vi "missing_Peak.vi"() -> ()   [LabVIEW 2016]
panel:
  out "x+y":i32
  out "Numeric":i32
  out "element":i32
  out "size(s)":i32
  out "Phase 2":dbl[](array[numeric])
  out "Peak Locations 2":i32[](array[numeric])
  in  "Width":dbl format="%#_13g"
  in  "Phase":dbl[](array[numeric])=[0.5, 1.55, 0.7, 0.8, 0.2, 0.3]
  in  "Peak Locations":i32[](array[numeric])=[1, 3, 4, 5]
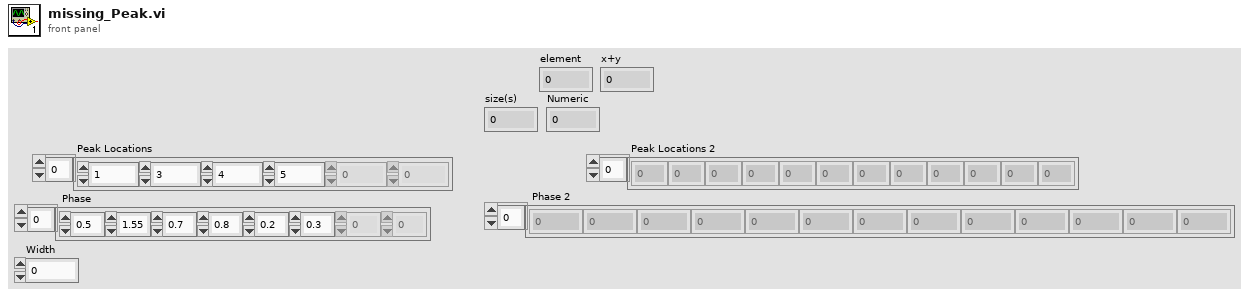
[diagram p1: front panel]
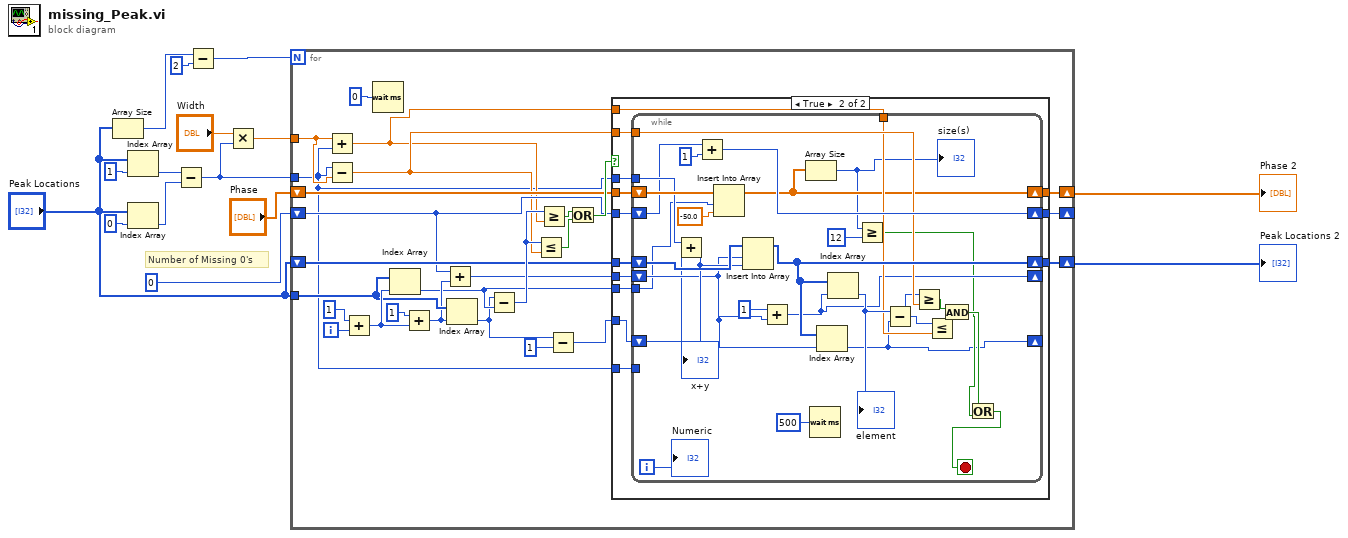
[diagram p0: block diagram]
diagram:
  # "Number of Missing 0's"
  n1 = Array Size(array="Peak Locations") -> (size(s)=w8:i32)
  n2 = Index Array(array="Peak Locations", index=1) -> (element=w13:i32)
  n3 = Index Array(array="Peak Locations", index=0) -> (element=w12:i32)
  n4 = Subtract(x=w13, y=w12) -> (x-y=w11:i32)
  n5 = Subtract(x=w8, y=2) -> (x-y=w6:i32)
  n6 = Multiply(x="Width", y=w11) -> (x*y=w9:dbl)
  n7 = for {
    N: w6 -> [_]
    tunnel: w11 -> [w16]
    tunnel: w9 -> [w20]
    shift-right: [w32] -> w4
    shift-left: "Phase" -> [w34]
    tunnel: "Peak Locations" -> [w30]
    shift-right: [w28] -> w2
    shift-left: "Peak Locations" -> [w29]
    shift-right: [w23] -> _
    shift-left: 0 -> [w24]
    i -> [w41]
    n8 = Add(x=w20, y=w16) -> (x+y=w21:dbl)
    n9 = Subtract(x=w16, y=w20) -> (x-y=w22:dbl)
    n10 = Add(x=1, y=w41) -> (x+y=w35:i32)
    n11 = Wait (ms)(milliseconds to wait=u32 0) -> ()  [unwired: 1 out]
    n12 = Index Array(array=w30, index=w35) -> (element=w25:i32)
    n13 = Add(x=1, y=w35) -> (x+y=w27:i32)
    n14 = Add(x=w24, y=w27) -> (x+y=w26:i32)
    n15 = Index Array(array=w30, index=w27) -> (element=w19:i32)
    n16 = Subtract(x=w19, y=w25) -> (x-y=w33:i32)
    n17 = Less Or Equal?(x=w33, y=w22) -> (x <= y?=w38:bool)
    n18 = Greater Or Equal?(x=w33, y=w21) -> (x >= y?=w37:bool)
    n19 = Subtract(x=w19, y=1) -> (x-y=w17:i32)
    n20 = Or(x=w37, y=w38) -> (x .or. y?=w36:bool)
    n21 = case shown="True" w36 {
      tunnel: w29 -> [w44 w57]
      tunnel: w26 -> [_ w56]
      tunnel: w34 -> [w43 w55]
      tunnel: w17 -> [_ w52]
      tunnel: [w44 w54] -> w28
      tunnel: [w43 w53] -> w32
      tunnel: w16 -> [_ w51]
      tunnel: w25 -> [_ w50]
      tunnel: w24 -> [w42 w49]
      tunnel: [w42 w48] -> w23
      tunnel: w22 -> [_ w47]
      tunnel: w21 -> [_ w46]
      tunnel: w16 -> [_ w45]
      frame False {
      }
      frame True {
        n22 = while {
          tunnel: w51 -> [w83]
          tunnel: w50 -> [w58]
          shift-right: [w79] -> w54
          shift-left: w57 -> [w86]
          shift-right: [w69] -> w53
          shift-left: w55 -> [w85]
          shift-right: [w80] -> w48
          shift-left: w49 -> [w82]
          tunnel: w47 -> [w72]
          tunnel: w46 -> [w71]
          shift-right: [w70] -> _
          shift-left: w56 -> [w75]
          shift-right: [w59] -> _
          shift-left: w52 -> [w60]
          tunnel: w45 -> [_]
          i -> [w66]
          stop <- w61 stop-if-true
          n23 = Add(x=w83, y=w60) -> (x+y=w78:i32)
          "x+y" <- w78
          n24 = Add(x=w82, y=1) -> (x+y=w80:i32)
          n25 = Insert Into Array(array=w85, index=w58, new element=-50.0 ("new element/subarray")) -> (w69:dbl[])
          n26 = Insert Into Array(array=w86, index=w75, new element=w78) -> (w79:i32[])
          n27 = Add(x=1, y=w75) -> (x+y=w70:i32)
          n28 = Array Size(array=w69) -> (size(s)=w64:i32)
          "size(s)" <- w64
          n29 = Wait (ms)(milliseconds to wait=u32 500) -> ()  [unwired: 1 out]
          n30 = Index Array(array=w79, index=w75) -> (element=w59:i32)
          n31 = Index Array(array=w79, index=w70) -> (element=w76:i32)
          "element" <- w76
          n32 = Greater Or Equal?(x=w64, y=12) -> (x >= y?=w62:bool)
          n33 = Subtract(x=w76, y=w59) -> (x-y=w67:i32)
          n34 = Greater Or Equal?(x=w67, y=w72) -> (x >= y?=w74:bool)
          n35 = Less Or Equal?(x=w67, y=w71) -> (x <= y?=w73:bool)
          n36 = And(x=w74, y=w73) -> (x .and. y?=w65:bool)
          n37 = Or(x=w65, y=w62) -> (x .or. y?=w61:bool)
          "Numeric" <- w66
        }
      }
    }
  }
  "Peak Locations 2" <- w2
  "Phase 2" <- w4
